vi "1 - Prepare Source Files.vi"() -> ()   [LabVIEW 2020]
panel:
  out "Processing":path
  out "error out":errorcluster
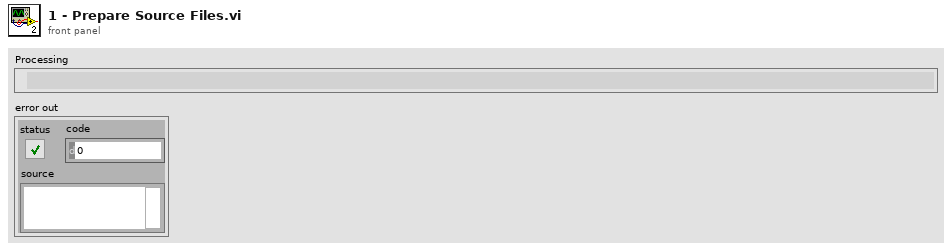
[diagram p1: front panel]
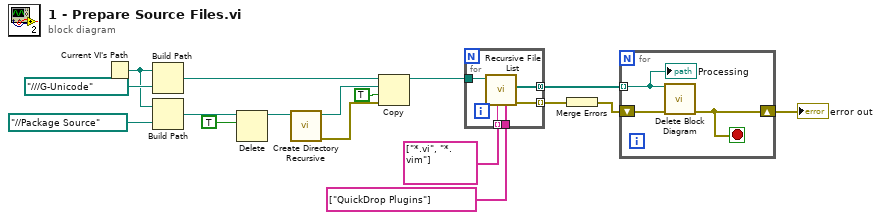
[diagram p0: block diagram]
diagram:
  n1 = Current VI's Path() -> (path=w15:path)
  n2 = Build Path(base path=w15, name or relative path=path "../../../G-Unicode") -> (appended path=w16:path)
  n3 = Build Path(base path=w15, name or relative path=path "../../Package Source") -> (appended path=w13:path)
  n4 = Delete(path (use dialog)=w13, entire hierarchy (F)=TRUE) -> (deleted path=w12:path)  [unwired: 3 in, 2 out]
  n5 = call <vilib>:"Create Directory Recursive.vi"("directory"=w12) -> ("error out"=w9:errorcluster, "directory copy"=w11:path)  [unwired: 4 in, 1 out]
  n6 = Copy(8:w9, 9:TRUE ("overwrite (F)"), 10:w11, 11:w16) -> (3:w7:path)  [unwired: 1 in, 2 out]
  n7 = for {
    tunnel: w7 -> [w22]
    tunnel: [w21] -> w5 mode=concatenating
    tunnel: string[] ["*.vi", "*.vim"] -> [w20] mode=indexing
    tunnel: [w19] -> w4 mode=indexing
    tunnel: string[] ["QuickDrop Plugins"] ("Folders to Exclude") -> [w18]
    n8 = call <vilib>:"Recursive File List.vi"("Folders to Exclude"=w18, "pattern"=w20, "Folder Path"=w22) -> ("error out"=w19:errorcluster, "All Files in Dir"=w21:path[])  [unwired: 4 in, 3 out]
  }
  n9 = Merge Errors(w4) -> (w3:errorcluster)
  n10 = for {
    tunnel: w5 -> [w25] mode=indexing
    shift-right: [w23] -> w2
    shift-left: w3 -> [w24]
    stop <- w23 stop-if-true
    n11 = call "Delete Block Diagram.vi"("error in (no error)"=w24, "VI Path"=w25) -> ("error out"=w23:errorcluster)  [unwired: 9 in]
    "Processing" <- w25
  }
  "error out" <- w2
